vi "ToDateTimeRec.vi"(0 "Time and Date":T2) -> (4 "Date Time Record":T1)   [LabVIEW 2017, in "GPTiming.lvlib"]
doc: "Converts a GPower <B>Time and Date</B> structure into a LabVIEW <B>Date Time Record</B>.\n\nSteen Schmidt\nGPower\n8/5 2016"
uses:
  GPTiming.lvlib
  <vilib>/Utility/miscctls.llb/LVDateTimeRec.ctl
  Date.ctl
  Time.ctl
  TimeAndDate.ctl
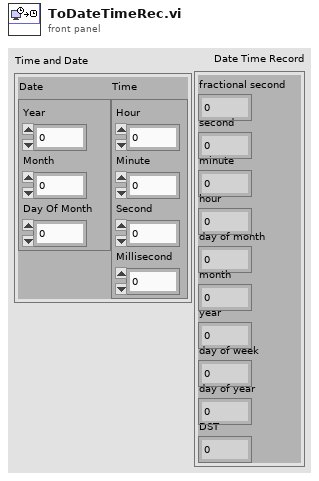
[diagram p1: front panel]
types:
  T1 = typedef "LVDateTimeRec.ctl" = cluster{"fractional second":dbl, "second":i32, "minute":i32, "hour":i32, "day of month":i32, "month":i32, "year":i32, "day of week":i32, "day of year":i32, "DST":i32}
  T2 = typedef "GPTiming.lvlib/TimeAndDate.ctl" = cluster{"Date":T3, "Time":T4}
  T3 = typedef "GPTiming.lvlib/Date.ctl" = cluster{"Year":u16, "Month":u16, "Day Of Month":u16}
  T4 = typedef "GPTiming.lvlib/Time.ctl" = cluster{"Hour":u16, "Minute":u16, "Second":u16, "Millisecond":u16}
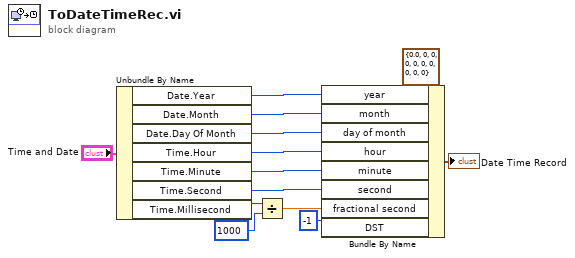
[diagram p0: block diagram]
diagram:
  n1 = Unbundle By Name("Time and Date") -> ("Date.Year"=w10:u16, "Date.Month"=w9:u16, "Date.Day Of Month"=w8:u16, "Time.Hour"=w7:u16, "Time.Minute"=w6:u16, "Time.Second"=w5:u16, "Time.Millisecond"=w4:u16)
  n2 = Divide(x=w4, y=u16 1000) -> (x/y=w2:dbl)
  n3 = Bundle By Name(cluster=T1 {"fractional second"=0.0, "second"=0, "minute"=0, "hour"=0, "day of month"=0, "month"=0, "year"=0, "day of week"=0, "day of year"=0, "DST"=0} ("date time rec"), "year"=w10, "month"=w9, "day of month"=w8, "hour"=w7, "minute"=w6, "second"=w5, "fractional second"=w2, "DST"=-1) -> (→"Date Time Record":T1)
